vi "test Log Archive.vi"(8 "error in (no error)":errorcluster, 11 "TestCase in":refnum<class "Embedded Data Logger System Tests.lvclass">) -> (0 "error out":errorcluster, 3 "TestCase out":refnum<class "Embedded Data Logger System Tests.lvclass">)   [LabVIEW 2018, in "Embedded Data Logger System Tests.lvclass"]
uses:
  Embedded Data Logger System Tests.lvclass
  <vilib>/addons/_JKI Toolkits/VI Tester/TestCase.llb/TestCase.lvclass
  C:/Program Files (x86)/National Instruments/LabVIEW 2018/vi.lib/addons/_JKI Toolkits/VI Tester/TestCase.llb/TestCase.lvclass
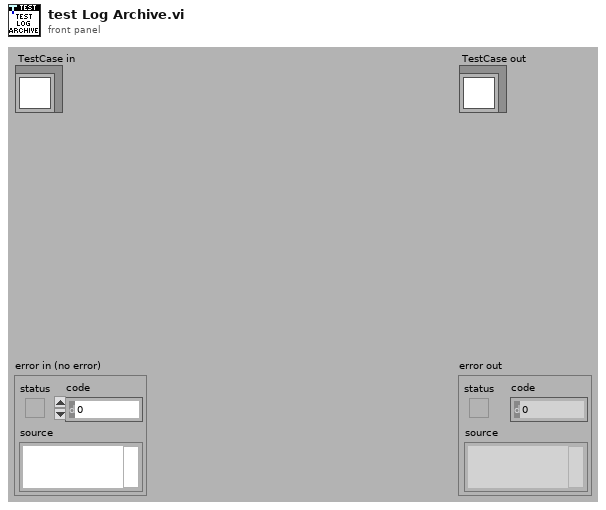
[diagram p1: front panel]
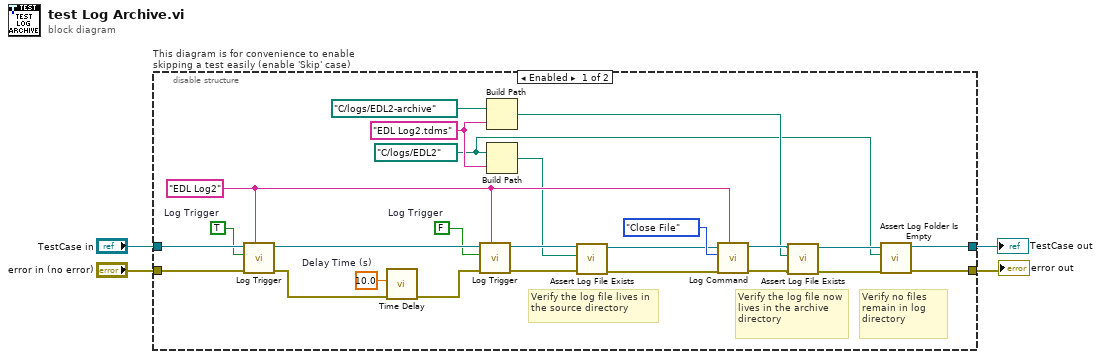
[diagram p0: block diagram]
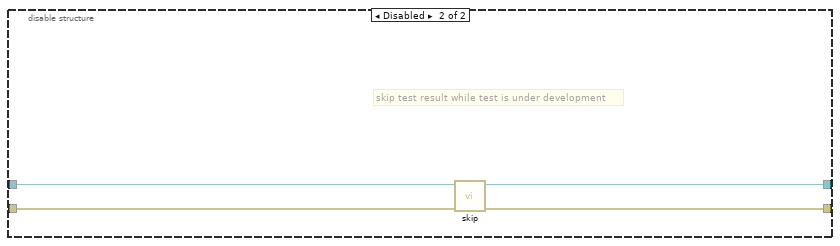
[diagram p2: hidden frame]
diagram:
  n1 = disable-structure "This diagram is for convenience to enable skipping a test easily (enable 'Skip' case)" shown="Enabled" {
    disable-tunnel: "TestCase in" -> [w29 w33]
    disable-tunnel: [w10 w31] -> w1
    disable-tunnel: [w11 w32] -> w3
    disable-tunnel: "error in (no error)" -> [w28 w30]
    frame Enabled {
      w8 = "EDL Log2.tdms" ("Embedded Data Logger File Name")
      w5 = path "C:/logs/EDL2" ("file path")
      w18 = "EDL Log2" ("Embedded Data Logger File Name")
      w22 = FALSE  # Log Trigger
      w23 = 10.0  # Delay Time (s)
      w25 = TRUE  # Log Trigger
      # "Verify no files remain in log directory"
      # "Verify the log file now lives in the archive directory"
      # "Verify the log file lives in the source directory"
      n2 = call "Log Trigger.vi"("Embedded Data Logger File Name"=w18, "error in"=w28, "Log Trigger"=w25, "Embedded Data Logger System Tests in"=w29) -> ("error out"=w26:errorcluster, "Embedded Data Logger System Tests out"=w27:refnum<class "Embedded Data Logger System Tests.lvclass">)  [unwired: 6 in]
      n3 = call "Time Delay"("error in (no error)"=w26, "Delay Time (s)"=w23) -> ("error out"=w24:errorcluster)  [unwired: 9 in]
      n4 = call "Log Trigger.vi"("Embedded Data Logger File Name"=w18, "error in"=w24, "Log Trigger"=w22, "Embedded Data Logger System Tests in"=w27) -> ("error out"=w16:errorcluster, "Embedded Data Logger System Tests out"=w17:refnum<class "Embedded Data Logger System Tests.lvclass">)  [unwired: 6 in]
      n5 = Build Path(base path=path "C:/logs/EDL2-archive" ("file path"), name or relative path=w8) -> (appended path=w6:path)
      n6 = Build Path(base path=w5, name or relative path=w8) -> (appended path=w7:path)
      n7 = call "Assert Log File Exists.vi"("error in"=w16, "file path"=w7, "Embedded Data Logger System Tests in"=w17) -> ("error out"=w14:errorcluster, "Embedded Data Logger System Tests out"=w15:refnum<class "Embedded Data Logger System Tests.lvclass">)  [unwired: 7 in]
      n8 = call "Log Command.vi"("Embedded Data Logger File Name"=w18, "error in"=w14, "Log Command"=enum16{"Idle", "Open File", "Close File"}."Close File", "Embedded Data Logger System Tests in"=w15) -> ("error out"=w19:errorcluster, "Embedded Data Logger System Tests out"=w20:refnum<class "Embedded Data Logger System Tests.lvclass">)  [unwired: 6 in]
      n9 = call "Assert Log File Exists.vi"("error in"=w19, "file path"=w6, "Embedded Data Logger System Tests in"=w20) -> ("error out"=w12:errorcluster, "Embedded Data Logger System Tests out"=w13:refnum<class "Embedded Data Logger System Tests.lvclass">)  [unwired: 7 in]
      n10 = call "Assert Log Folder Is Empty.vi"("error in"=w12, "directory"=w5, "Embedded Data Logger System Tests in"=w13) -> ("error out"=w11:errorcluster, "Embedded Data Logger System Tests out"=w10:refnum<class "Embedded Data Logger System Tests.lvclass">)  [unwired: 7 in]
    }
    frame Disabled {
      # "skip test result while test is under development"
      n11 = call <vilib>:"skip.vi"("error in (no error)"=w30, "TestCase in"=w33) -> ("error out"=w32:errorcluster, "TestCase out"=w31:refnum<class "Embedded Data Logger System Tests.lvclass">)  [unwired: 8 in]
    }
  }
  "error out" <- w3
  "TestCase out" <- w1
